vi "Determine Database Change List.vi"(8 "error in (no error)":errorcluster, 10 "Old Cluster":refnum<k21>="NI_Support_20250912", 11 "New Cluster":refnum<k21>="NI_Support_20250912_New") -> (0 "error out":errorcluster, 3 "XNET Change List":T1)   [LabVIEW 2025, in "Protection and Counter Addon System Explorer.lvlib"]
uses:
  Protection and Counter Addon System Explorer.lvlib
  Types/XNET Change List.ctl
  Types/Base Frame Info_NoVS.ctl
  Types/Signal Attributes.ctl
  Types/CAN Filter Type.ctl
  Types/Related CAN Frames No VS.ctl
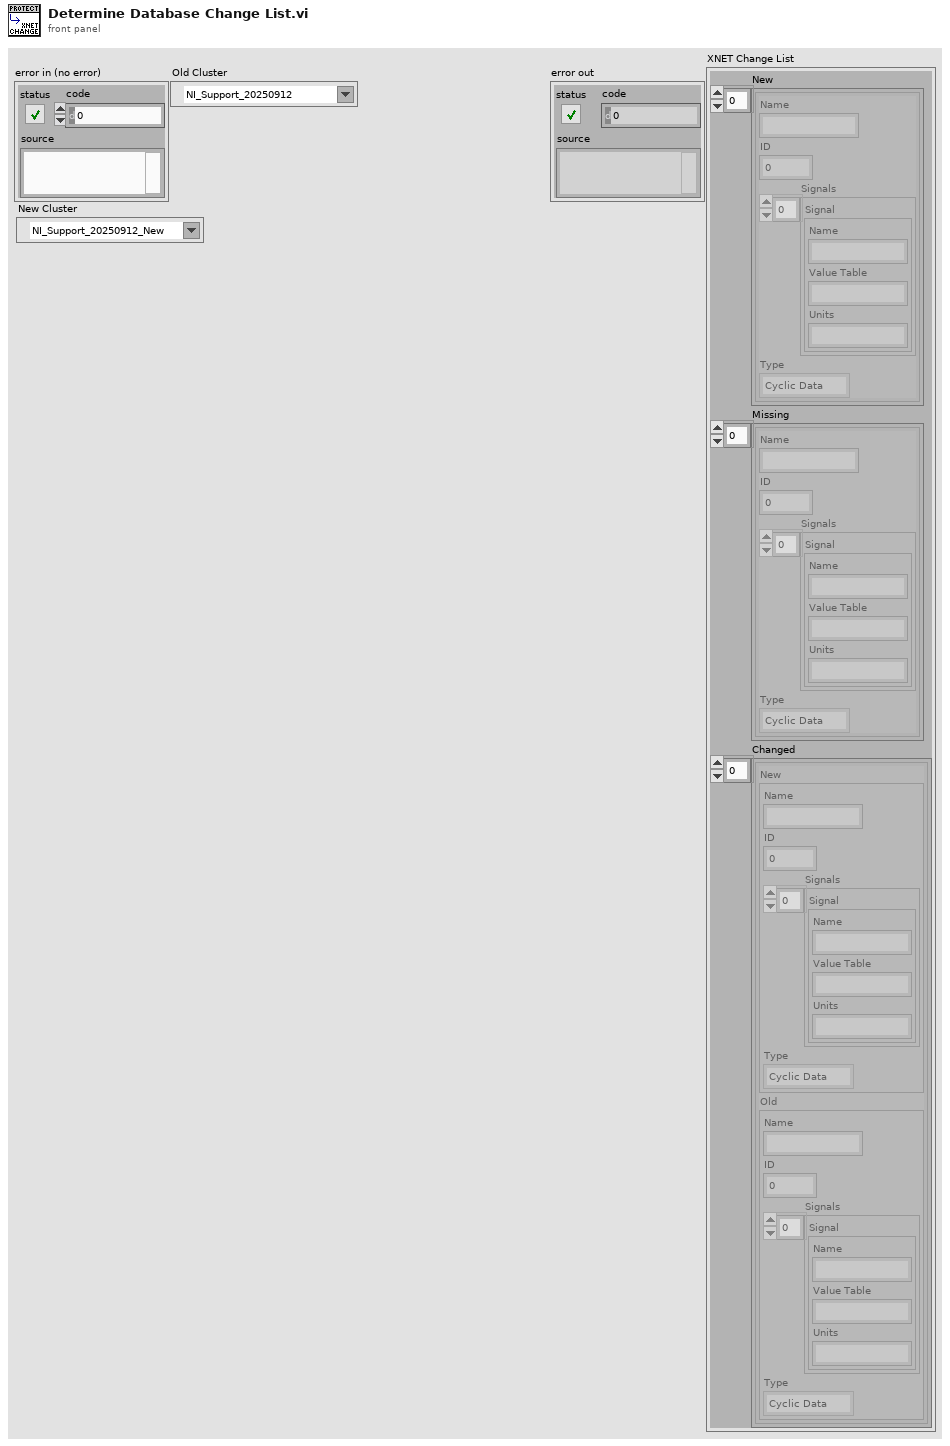
[diagram p1: front panel]
types:
  T1 = typedef "Protection and Counter Addon System Explorer.lvlib/XNET Change List.ctl" = cluster{"New":T2[], "Missing":T2[], "Changed":T5[]}
  T2 = typedef "Protection and Counter Addon System Explorer.lvlib/Base Frame Info_NoVS.ctl" = cluster{"Name":string, "ID":u32, "Signals":T3[], "Type":T4}
  T3 = typedef "Protection and Counter Addon System Explorer.lvlib/Signal Attributes.ctl" = cluster{"Name":string, "Value Table":string, "Units":string}
  T4 = typedef "Protection and Counter Addon System Explorer.lvlib/CAN Filter Type.ctl" = enum16{"Cyclic Data", "Event Data", "Cyclic/Event", "All"}
  T5 = typedef "Protection and Counter Addon System Explorer.lvlib/Related CAN Frames No VS.ctl" = cluster{"New":T2, "Old":T2}
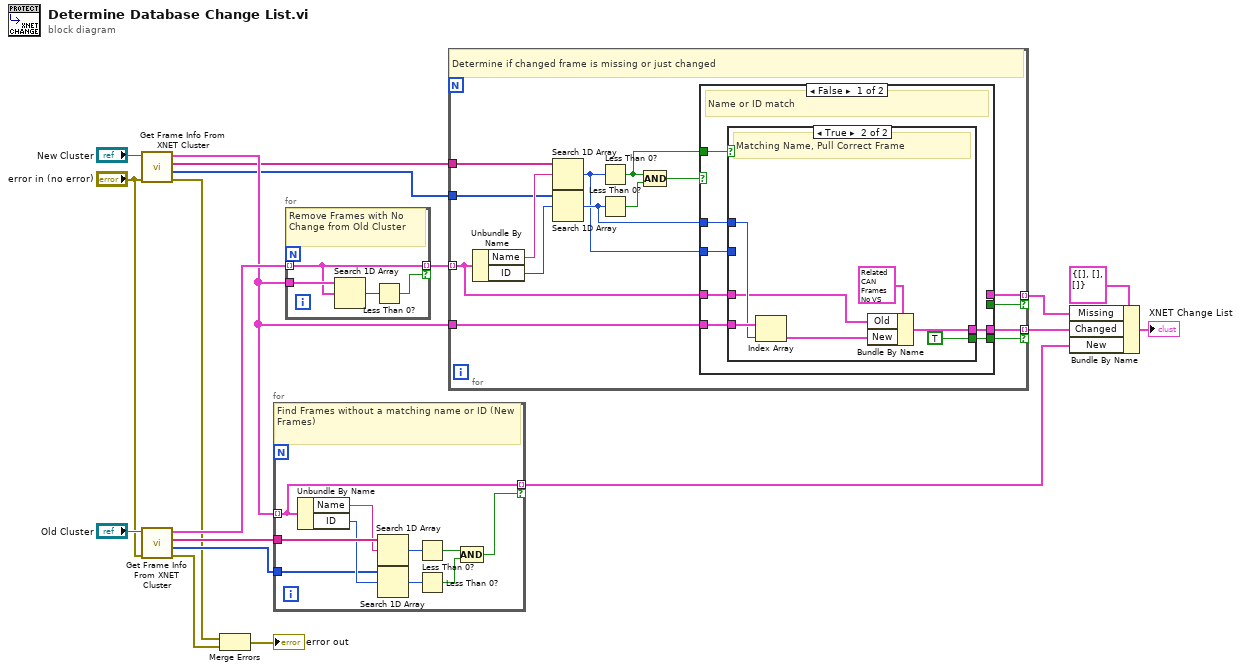
[diagram p0: block diagram]
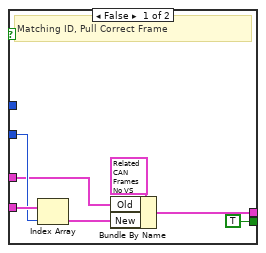
[diagram p2: hidden frame]
diagram:
  n1 = call "Get Frame Info From XNET Cluster.vi"("error in (no error)"="error in (no error)", "Cluster In"="New Cluster") -> ("error out"=w7:errorcluster, "Frame IDs"=w9:u32[], "Frame Names"=w8:string[], "Frame Info"=w10:T2[])  [unwired: 6 in]
  n2 = call "Get Frame Info From XNET Cluster.vi"("error in (no error)"="error in (no error)", "Cluster In"="Old Cluster") -> ("error out"=w17:errorcluster, "Frame IDs"=w14:u32[], "Frame Names"=w15:string[], "Frame Info"=w13:T2[])  [unwired: 6 in]
  n3 = Merge Errors(w7, w17) -> (→"error out":errorcluster)
  n4 = for {
    tunnel: w10 -> [w20] mode=indexing
    tunnel: w15 -> [w28]
    tunnel: w14 -> [w25]
    tunnel: [w20] -> w3 mode=indexing if=w19
    # "Find Frames without a matching name or ID (New Frames)"
    n5 = Unbundle By Name(w20) -> ("Name"=w27:string, "ID"=w26:u32)
    n6 = Search 1D Array(1D array=w28, element=w27) -> (index of element=w24:i32)  [unwired: 1 in]
    n7 = Search 1D Array(1D array=w25, element=w26) -> (index of element=w23:i32)  [unwired: 1 in]
    n8 = Less Than 0?(x=w24) -> (x < 0?=w22:bool)
    n9 = Less Than 0?(x=w23) -> (x < 0?=w21:bool)
    n10 = Compound Arithmetic op=AND(w22, w21) -> (w19:bool)
  }
  n11 = for {
    tunnel: w10 -> [w32]
    tunnel: w13 -> [w30] mode=indexing
    tunnel: [w30] -> w12 mode=indexing if=w29
    # "Remove Frames with No Change from Old Cluster"
    n12 = Search 1D Array(1D array=w32, element=w30) -> (index of element=w31:i32)  [unwired: 1 in]
    n13 = Less Than 0?(x=w31) -> (x < 0?=w29:bool)
  }
  n14 = for {
    tunnel: w12 -> [w41] mode=indexing
    tunnel: w8 -> [w47]
    tunnel: w9 -> [w44]
    tunnel: [w40] -> w5 mode=indexing if=w39
    tunnel: w10 -> [w37]
    tunnel: [w34] -> w4 mode=indexing if=w33
    # "Determine if changed frame is missing or just changed"
    n15 = Unbundle By Name(w41) -> ("Name"=w46:string, "ID"=w45:u32)
    n16 = Search 1D Array(1D array=w47, element=w46) -> (index of element=w35:i32)  [unwired: 1 in]
    n17 = Search 1D Array(1D array=w44, element=w45) -> (index of element=w36:i32)  [unwired: 1 in]
    n18 = Less Than 0?(x=w35) -> (x < 0?=w38:bool)
    n19 = Less Than 0?(x=w36) -> (x < 0?=w43:bool)
    n20 = Compound Arithmetic op=AND(w38, w43) -> (w42:bool)
    n21 = case shown="False" w42 {
      selector: w42 -> [_ w69]
      tunnel: w41 -> [w50 w70]
      tunnel: [_ w70] -> w40
      tunnel: [_ w69] -> w39
      tunnel: w38 -> [w54 _]
      tunnel: w37 -> [w53 _]
      tunnel: w36 -> [w52 _]
      tunnel: w35 -> [w51 _]
      tunnel: [w49 _] -> w34
      tunnel: [w48 _] -> w33
      frame False {
        # "Name or ID match"
        n22 = case shown="True" w54 {
          tunnel: w53 -> [w61 w68]
          tunnel: w52 -> [_ w67]
          tunnel: w51 -> [w60 _]
          tunnel: w50 -> [w56 w64]
          tunnel: [w55 w63] -> w49
          tunnel: [TRUE TRUE] -> w48
          frame False {
            # "Matching ID, Pull Correct Frame"
            n23 = Index Array(array=w61, index=w60) -> (element=w57:T2)
            n24 = Bundle By Name(cluster=T5 {"New"={"Name"="", "ID"=0, "Signals"=[], "Type"=enum."Cyclic Data"}, "Old"={"Name"="", "ID"=0, "Signals"=[], "Type"=enum."Cyclic Data"}}, "Old"=w56, "New"=w57) -> (w55:T5)
          }
          frame True {
            # "Matching Name, Pull Correct Frame"
            n25 = Index Array(array=w68, index=w67) -> (element=w65:T2)
            n26 = Bundle By Name(cluster=T5 {"New"={"Name"="", "ID"=0, "Signals"=[], "Type"=enum."Cyclic Data"}, "Old"={"Name"="", "ID"=0, "Signals"=[], "Type"=enum."Cyclic Data"}}, "Old"=w64, "New"=w65) -> (w63:T5)
          }
        }
      }
      frame True {
        # "No matching Name and no matching ID = Missing"
      }
    }
  }
  n27 = Bundle By Name(cluster=T1 {"New"=[], "Missing"=[], "Changed"=[]}, "Missing"=w5, "Changed"=w4, "New"=w3) -> (→"XNET Change List":T1)
